vi "Actor Core.vi"(8 "error in (no error)":errorcluster, 11 "Operator UI.lvclass":refnum<class "Measurement Setup UI.lvclass">) -> (0 "error out":errorcluster, 3 "Actor Framework.lvlib:Actor":refnum<class "Actor.lvclass">)   [LabVIEW 2016, in "Measurement Setup Controller.lvlib" / "Measurement Setup UI.lvclass"]
doc: "This is Actor Core.vi, the main message handling loop for Actors. An actor usually just sits in this loop and processes messages as they arrive. Any error returned by the message Do.vi call will stop the loop, with error code 43 as the cannonical signal to stop with no error sent to caller. Descendants may override that in Handle Error.vi."
uses:
  Measurement Setup UI.lvclass
  <vilib>/ActorFramework/Actor/Actor.lvclass
  \\Mac\Home/Documents/MAL-Framework/user.lib/Common Components/Msmt UI/Measurement UI.lvclass
  \\Mac\Home/Documents/MAL-Framework/user.lib/Common Components/User Interface/UI.lvclass
  C:/Program Files (x86)/National Instruments/LabVIEW 2016/vi.lib/ActorFramework/Actor/Actor.lvclass
  Measurement Setup UI.lvclass/Measurement Setup UI.ctl
  <vilib>/ActorFramework/Actor/Actor.lvclass/Actor.ctl
  <vilib>/ActorFramework/Message Enqueuer/Message Enqueuer.lvclass/Message Enqueuer.ctl
  Write Save.vi
  <vilib>/ActorFramework/Message Enqueuer/Init from Existing Queue.vi
  <vilib>/ActorFramework/Message Enqueuer/Enqueue.vi
  <vilib>/ActorFramework/Stop Msg/Stop Msg.lvclass
  C:/Program Files (x86)/National Instruments/LabVIEW 2016/vi.lib/ActorFramework/Message/Message.lvclass
  Measurement Setup UI Messages/Save Configuration Msg/Save Configuration Msg.lvclass
  MAL-Framework/user.lib/Common Components/Msmt UI/Messages/Ask Controller to Launch Results UI Msg/Ask Controller to Launch Results UI Msg.lvclass
  MAL-Framework/user.lib/Common Components/Measurement UI Messages/Launch Step Configuration Msg/Launch Step Configuration Msg.lvclass
  MAL-Framework/user.lib/Common Components/Msmt UI/Accessors/Write Digitizer.vi
  MAL-Framework/user.lib/Common Components/Msmt UI/Accessors/Write Function Generator.vi
  MAL-Framework/user.lib/Common Components/Msmt UI/Accessors/Write Measurement.vi
  MAL-Framework/user.lib/Common Components/Msmt UI/Accessors/Write Multimeter.vi
  MAL-Framework/user.lib/Common Components/Msmt UI/Accessors/Write Power Supply.vi
  MAL-Framework/user.lib/Common Components/Msmt UI/Accessors/Write Results Listbox.vi
  MAL-Framework/user.lib/Common Components/Msmt UI/Accessors/Write Run.vi
  MAL-Framework/user.lib/Common Components/Msmt UI/Accessors/Write Show FP_.vi
  MAL-Framework/user.lib/Common Components/Msmt UI/Accessors/Write Status Display.vi
  MAL-Framework/user.lib/Common Components/Msmt UI/Accessors/Write Tab Control.vi
  MAL-Framework/user.lib/Common Components/Msmt UI/Accessors/Write View Results.vi
  MAL-Framework/user.lib/Common Components/Msmt UI/Write settings button array for hardware.vi
  MAL-Framework/user.lib/Common Components/Msmt UI/Accessors/Write Step Config.vi
  <vilib>/ActorFramework/Message Priority Queue/Priority Enqueue.vi
  <vilib>/ActorFramework/Message Enqueuer/Message Enqueuer.lvclass
  MAL-Framework/user.lib/Common Components/Msmt UI/Measurement UI.lvclass
  MAL-Framework/user.lib/Common Components/Msmt UI/Messages/Send Run Measurement Message/Send Run Measurement Message.lvclass
  MAL-Framework/user.lib/Common Components/Msmt UI/Messages/Send Get Hardware Info Message/Send Get Hardware Info Message.lvclass
  MAL-Framework/user.lib/Common Components/Msmt UI/Messages/Check Run Button/Check Validity of Selection.lvclass
  MAL-Framework/user.lib/Common Components/User Interface/UI.lvclass
  MAL-Framework/user.lib/Common Components/Measurement UI Messages/Launch Hardware Settings Msg/Launch Hardware Settings Msg.lvclass
panel:
  in  "Step Config":bool
  in  "3":bool
  in  "2":bool
  in  "1":bool
  in  "0":bool
  in  "Cancel Button":bool
  in  "Save Button":bool
  in  "about":bool
  in  "Run":bool
  in  "Show FP?":bool
  in  "Power Supply":u16(ring) caption="Device 4"
  in  "Function Generator":u16(ring) caption="Device 3"
  in  "Digitizer":u16(ring) caption="Device 2"
  in  "Multimeter":u16(ring) caption="Device 1"
  in  "Tab Control":enum32{"Test Status", "Results"}(tab)
  in  "Status Display":string
  in  "View Results":bool
  in  "Results Listbox":i32(listbox)
  in  "Measurement":u16(ring)
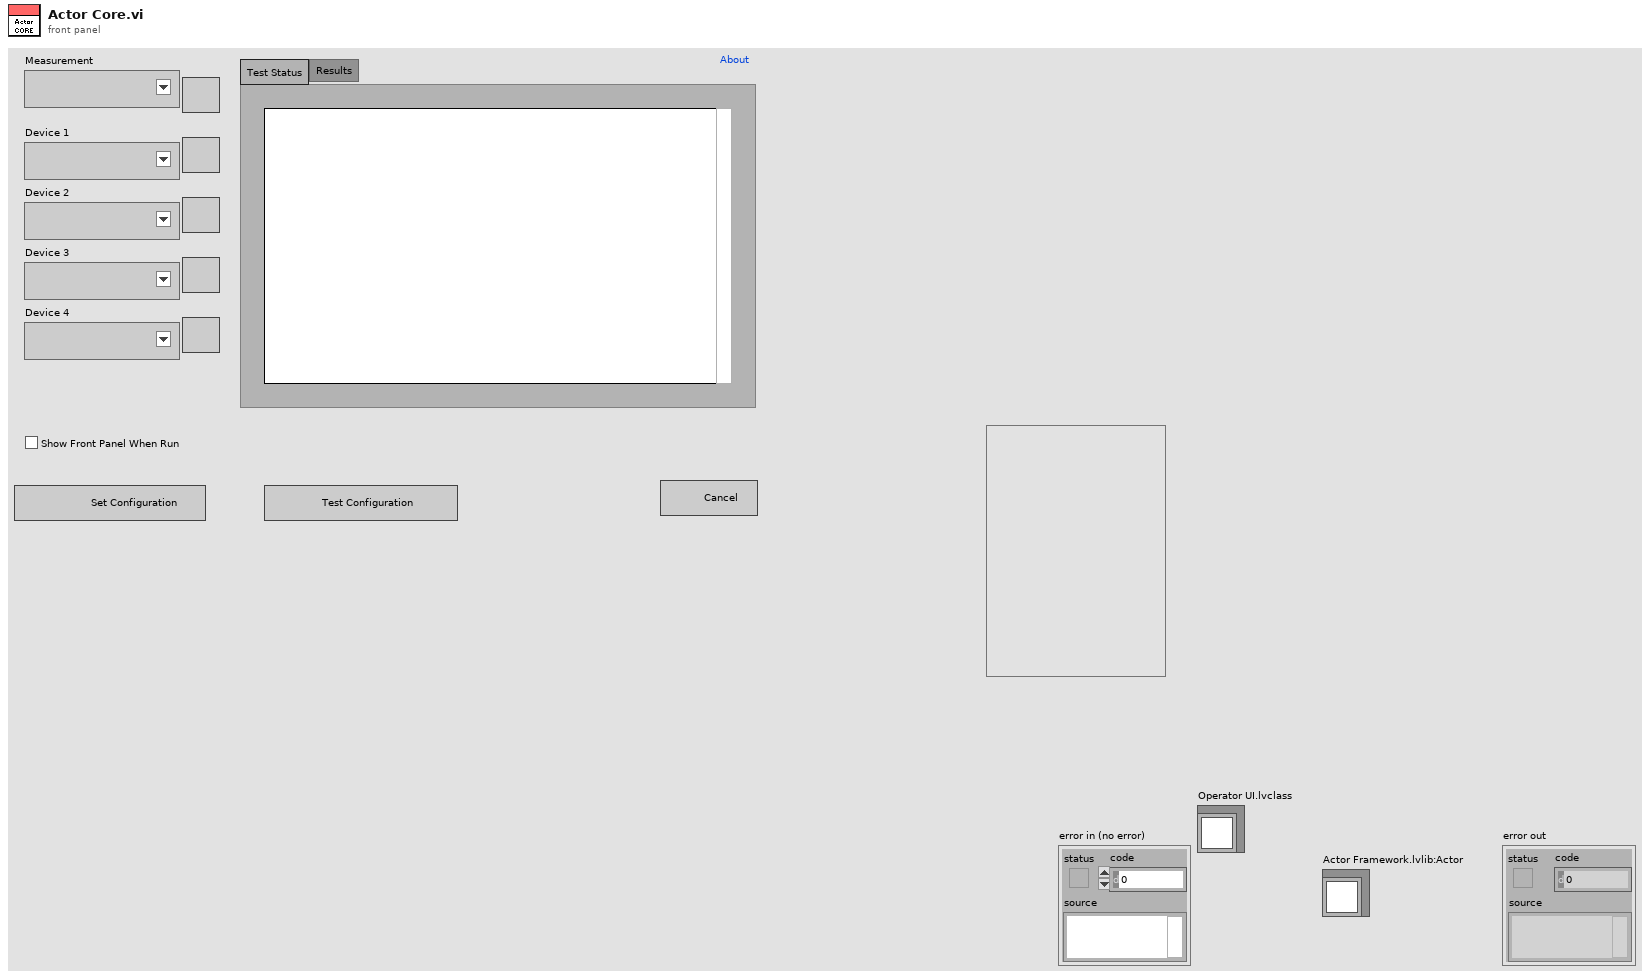
[diagram p1: front panel]
types:
  T1 = enum8{"Enabled", "Disabled", "Disabled and Grayed Out"}
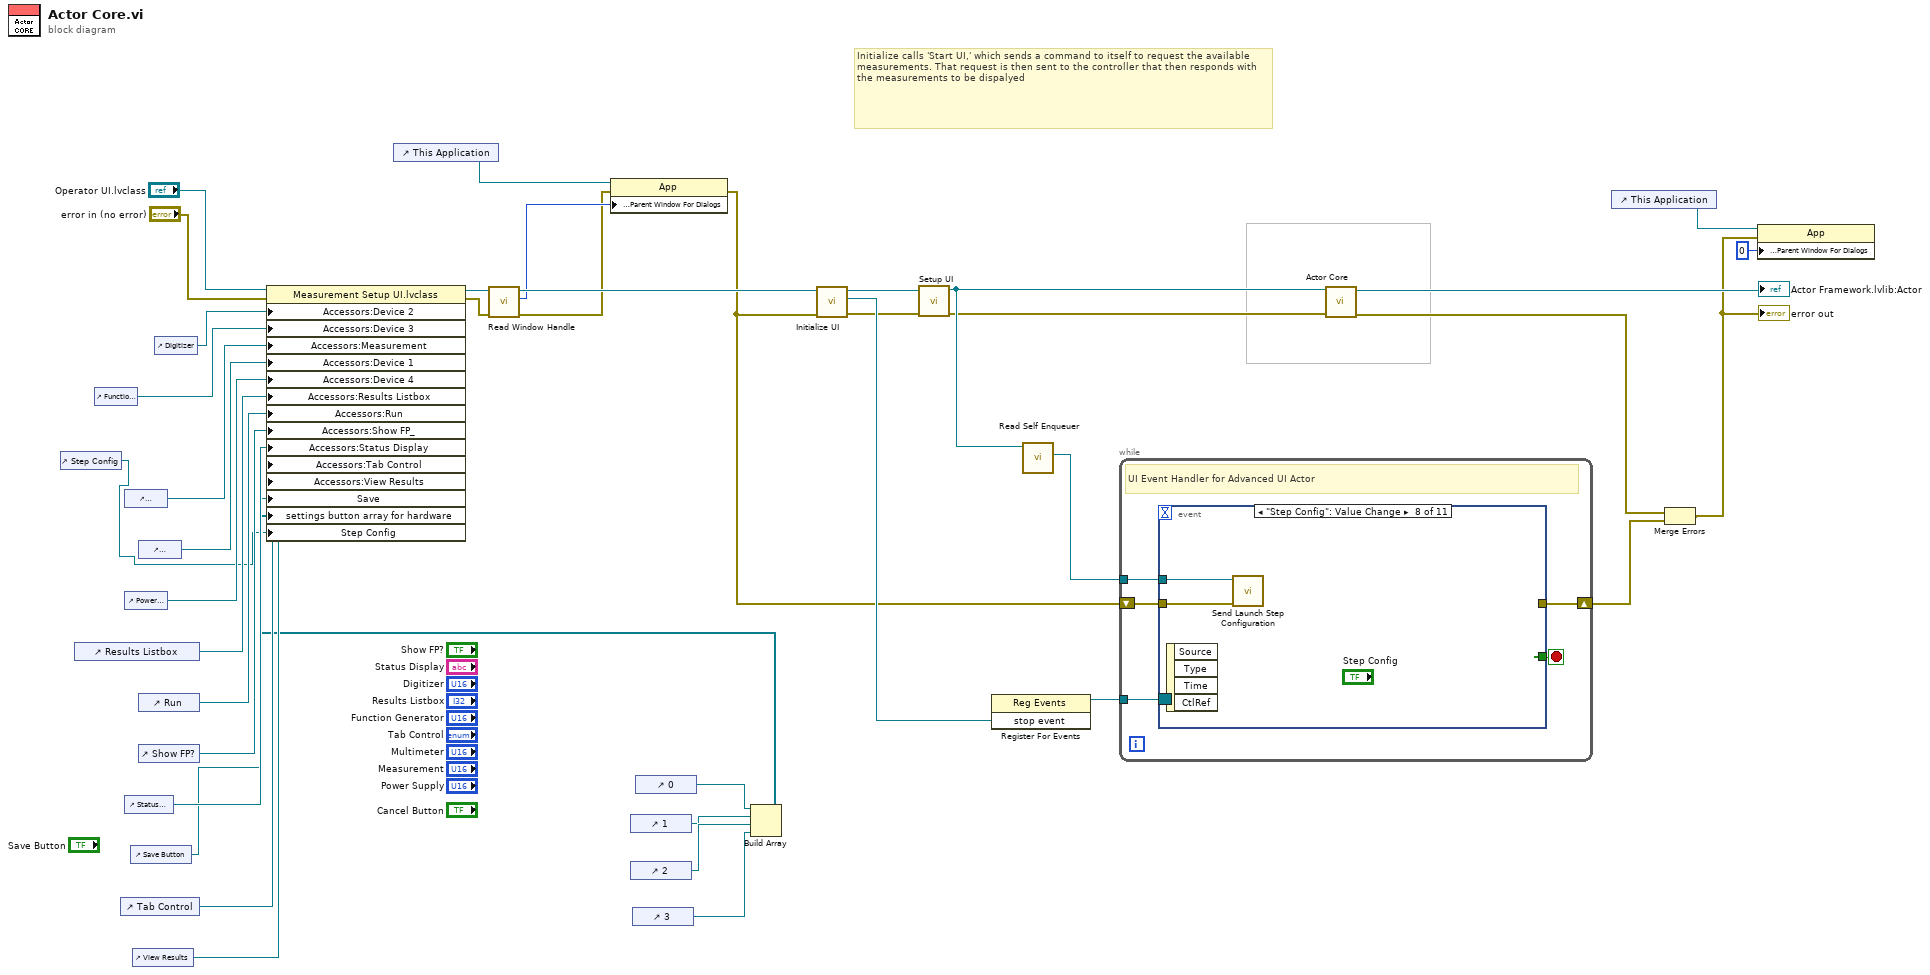
[diagram p0: block diagram]
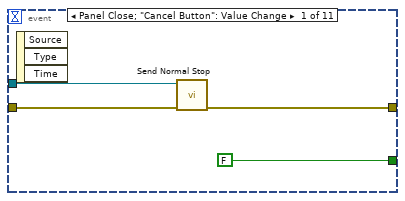
[diagram p2: hidden frame]
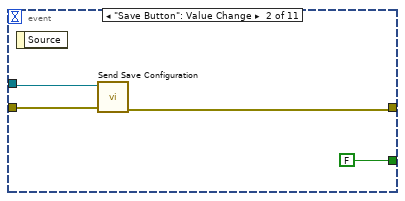
[diagram p3: hidden frame]
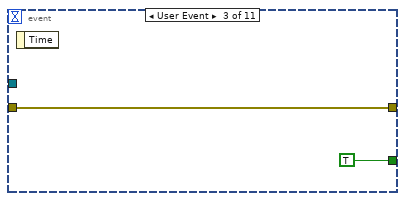
[diagram p4: hidden frame]
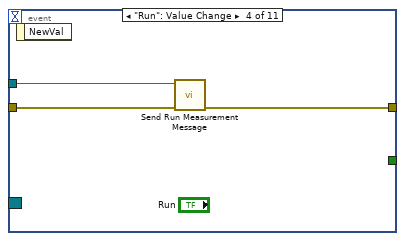
[diagram p5: hidden frame]
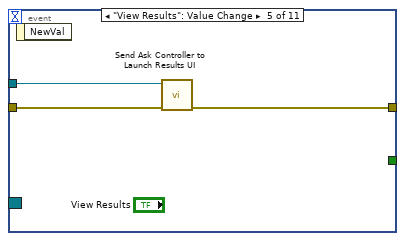
[diagram p6: hidden frame]
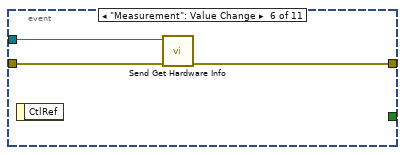
[diagram p7: hidden frame]
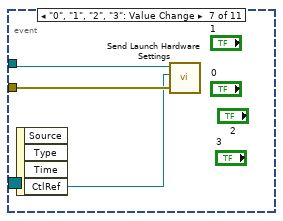
[diagram p8: hidden frame]
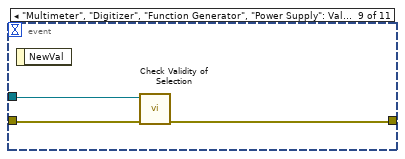
[diagram p9: hidden frame]
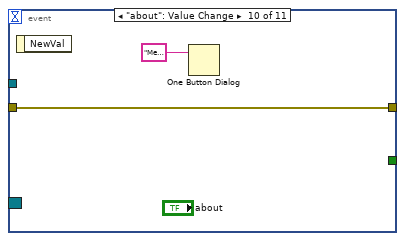
[diagram p10: hidden frame]
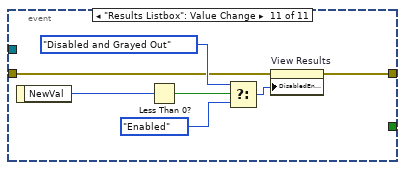
[diagram p11: hidden frame]
diagram:
  # "Initialize calls 'Start UI,' which sends a command to itself to request the available measurements. That request is then sent to the controller that then responds with the measurements to be dispalyed"
  n1 = control-ref of="Step Config"() -> (w1:refnum<vi>)
  n2 = control-ref of="Results Listbox"() -> (w31:refnum<vi>)
  n3 = control-ref of="Function Generator"() -> (w28:refnum<vi>)
  n4 = control-ref of="Tab Control"() -> (w33:refnum<vi>)
  n5 = control-ref of="Measurement"() -> (w27:refnum<vi>)
  n6 = control-ref of="Power Supply"() -> (w30:refnum<vi>)
  n7 = control-ref of="Status Display"() -> (w34:refnum<vi>)
  n8 = control-ref of="Save Button"() -> (w16:refnum<vi>)
  n9 = control-ref of="View Results"() -> (w32:refnum<vi>)
  n10 = control-ref of="Multimeter"() -> (w26:refnum<vi>)
  n11 = control-ref of="Run"() -> (w25:refnum<vi>)
  n12 = control-ref of="Show FP?"() -> (w35:refnum<vi>)
  n13 = control-ref of="Digitizer"() -> (w29:refnum<vi>)
  n14 = control-ref of="This Application"() -> (w12:refnum<vi>)
  n15 = control-ref of="1"() -> (w4:refnum<vi>)
  n16 = control-ref of="2"() -> (w5:refnum<vi>)
  n17 = control-ref of="3"() -> (w6:refnum<vi>)
  n18 = control-ref of="0"() -> (w3:refnum<vi>)
  n19 = Build Array(w3, w4, w5, w6) -> (w2:refnum<vi>[])
  n20 = property class="Measurement Setup UI.lvclass"(reference="Operator UI.lvclass", error in="error in (no error)", "Accessors:Device 2"=w29, "Accessors:Device 3"=w28, "Accessors:Measurement"=w27, "Accessors:Device 1"=w26, "Accessors:Device 4"=w30, "Accessors:Results Listbox"=w31, "Accessors:Run"=w25, "Accessors:Show FP_"=w35, "Accessors:Status Display"=w34, "Accessors:Tab Control"=w33, "Accessors:View Results"=w32, "Save"=w16, "settings button array for hardware"=w2, "Step Config"=w1) -> (reference out=w24:refnum<class "Measurement Setup UI.lvclass">, error out=w14:errorcluster)
  n21 = call "Read Window Handle.vi"("error in (no error)"=w14, "Measurement Setup UI in"=w24) -> ("error out"=w8:errorcluster, "Window Handle"=w13:i32, "Measurement Setup UI out"=w15:refnum<class "Measurement Setup UI.lvclass">)  [unwired: 7 in]
  n22 = property class="App"(reference=w12, error in=w8, "Application:Parent Window For Dialogs"=w13) -> (error out=w7:errorcluster)  [unwired: 1 out]
  n23 = call "Initialize UI.vi"("error in (no error)"=w7, "UI in"=w15) -> ("error out"=w22:errorcluster, "stop event"=w36:refnum<user-event>, "UI out"=w23:refnum<class "Measurement Setup UI.lvclass">)  [unwired: 7 in]
  n24 = call-dynamic "Setup UI.vi"("error in (no error)"=w22, "Operator UI in"=w23) -> ("error out"=w20:errorcluster, "Operator UI out"=w21:refnum<class "Measurement Setup UI.lvclass">)  [unwired: 8 in]
  n25 = register-events(w36) -> (reference out=w37:refnum<event-registration>)  [unwired: 2 in, 1 out]
  n26 = call <vilib>:"Read Self Enqueuer.vi"("Actor"=w21) -> ("Self Enqueuer"=w40:refnum<class "Message Enqueuer.lvclass">)  [unwired: 10 in]
  n27 = while {
    tunnel: w40 -> [w44]
    tunnel: w37 -> [w43]
    shift-right: [w41] -> w39
    shift-left: w7 -> [w42]
    stop <- w45 stop-if-true
    # "UI Event Handler for Advanced UI Actor"
    n28 = event shown="[7] \"Step Config\": Value Change" {
      selector: w43 -> [_ _ _ _ _ _ _ _ _ _ _]
      dyn-events: _ -> [_ _ _ _ _ _ _ _ _ _ _]
      timeout: _ -> [_ _ _ _ _ _ _ _ _ _ _]
      tunnel: [FALSE FALSE TRUE _ _ _ _ _ _ _ _] -> w45
      tunnel: w44 -> [w48 w53 _ w58 w61 w64 w67 w69 w72 _ _]
      tunnel: w42 -> [w47 w52 w54 w57 w60 w63 w66 w68 w71 w73 w76]
      tunnel: [w46 w51 w54 w56 w59 w62 _ _ w70 w73 w75] -> w41
      event Panel Close; "Cancel Button": Value Change {
        n29 = event-data() -> ()  [unwired: 1 in, 3 out]
        n30 = call <vilib>:"Send Normal Stop.vi"("error in (no error)"=w47, "Message Enqueuer"=w48) -> ("error out"=w46:errorcluster)  [unwired: 9 in]
      }
      event "Save Button": Value Change {
        n31 = event-data() -> ()  [unwired: 1 in, 1 out]
        n32 = call "Send Save Configuration.vi"("error in (no error)"=w52, "Message Enqueuer"=w53) -> ("error out"=w51:errorcluster)  [unwired: 8 in, 1 out]
      }
      event User Event {
        n33 = event-data() -> ()  [unwired: 1 in, 1 out]
      }
      event "Run": Value Change {
        n34 = event-data() -> ()  [unwired: 1 in, 1 out]
        n35 = call "Send Run Measurement Message.vi"("error in (no error)"=w57, "Message Enqueuer in"=w58) -> ("error out"=w56:errorcluster)  [unwired: 8 in, 1 out]
      }
      event "View Results": Value Change {
        n36 = event-data() -> ()  [unwired: 1 in, 1 out]
        n37 = call "Send Ask Controller to Launch Results UI.vi"("error in (no error)"=w60, "Message Enqueuer in"=w61) -> ("error out"=w59:errorcluster)  [unwired: 8 in, 1 out]
      }
      event "Measurement": Value Change {
        n38 = event-data() -> ()  [unwired: 1 in, 1 out]
        n39 = call "Send Get Hardware Info.vi"("error in (no error)"=w63, "Message Enqueuer in"=w64) -> ("error out"=w62:errorcluster)  [unwired: 8 in, 1 out]
      }
      event "0", "1", "2", "3": Value Change {
        n40 = event-data() -> ("CtlRef"=w65:refnum<vi>)  [unwired: 1 in, 3 out]
        n41 = call "Send Launch Hardware Settings.vi"("error in (no error)"=w66, "button ref"=w65, "Message Enqueuer"=w67) -> ()  [unwired: 7 in, 2 out]
      }
      event "Step Config": Value Change {
        n42 = event-data() -> ()  [unwired: 1 in, 4 out]
        n43 = call "Send Launch Step Configuration.vi"("error in (no error)"=w68, "Message Enqueuer"=w69) -> ()  [unwired: 8 in, 2 out]
      }
      event "Multimeter", "Digitizer", "Function Generator", "Power Supply": Value Change {
        n44 = event-data() -> ()  [unwired: 1 in, 1 out]
        n45 = call "Check Validity of Selection.vi"("error in (no error)"=w71, "Message Enqueuer in"=w72) -> ("error out"=w70:errorcluster)  [unwired: 8 in, 1 out]
      }
      event "about": Value Change {
        n46 = event-data() -> ()  [unwired: 1 in, 1 out]
        n47 = One Button Dialog(message="Measurement Configuration Utility\n\nNational Instruments (C) 2013\nWritten in NI LabVIEW 2013 by Elijah Kerry \nElijah.Kerry@ni.com\n\nni.com/largeapps\nekerry.wordpress.com") -> ()  [unwired: 1 in, 1 out]
      }
      event "Results Listbox": Value Change {
        n48 = event-data() -> ("NewVal"=w77:i32)  [unwired: 1 in]
        n49 = Less Than 0?(x=w77) -> (x < 0?=w78:bool)
        n50 = Select(t=T1."Disabled and Grayed Out" ("Disabled"), s=w78, f=T1."Enabled" ("Disabled")) -> (s? t:f=w81:T1)
        n51 = property on="View Results" class="Bool"(error in=w76, "DisabledEnum"=w81) -> (error out=w75:errorcluster)  [unwired: 1 in, 1 out]
      }
    }
  }
  n52 = call-parent "Actor Core.vi"("error in (no error)"=w20, "Operator UI.lvclass"=w21) -> ("error out"=w38:errorcluster, "Actor Framework.lvlib:Actor"=→"Actor Framework.lvlib:Actor":refnum<class "Actor.lvclass">)  [unwired: 8 in]
  n53 = control-ref of="This Application"() -> (w11:refnum<vi>)
  n54 = Merge Errors(w38, w39) -> (w10:errorcluster)
  "error out" <- w10
  n55 = property class="App"(reference=w11, error in=w10, "Application:Parent Window For Dialogs"=0) -> ()  [unwired: 2 out]
